vi "ControlClass.vi"(7 "PythonConverter_GUI in":refnum<class "PythonConverter_GUI.lvclass">, 8 "error in":errorcluster, 11 "Control in":refnum<class "Control.lvclass">) -> (0 "error out":errorcluster, 3 "Control out":refnum<class "Control.lvclass">, 4 "control name":string, 5 "PythonConverter_GUI out":refnum<class "PythonConverter_GUI.lvclass">)   [LabVIEW 2014, in "Raspberry Pi Compatible Compiler for LabVIEW.lvlib" / "PythonConverter_GUI.lvclass"]
uses:
  PythonConverter_GUI.lvclass
  VI Interpreter/Classes/Control/Control.lvclass
  VI Interpreter/Classes/NumericWithScale/NumericWithScale.lvclass/NumericWithScale.ctl
  Parsing/ClassTypeTD.ctl
  VI Interpreter/Classes/Control/Control.lvclass/Control.ctl
  VI Interpreter/Classes/Digital/Digital.lvclass
  VI Interpreter/Classes/Tab/Tab.lvclass
  VI Interpreter/Classes/Cluster/Cluster.lvclass
  VI Interpreter/Classes/Knob/Knob.lvclass
  VI Interpreter/Classes/Slide/Slide.lvclass
  VI Interpreter/Classes/Ring/Ring.lvclass
  VI Interpreter/Classes/Enum/Enum.lvclass
  VI Interpreter/Classes/NumericWithScale/NumericWithScale.lvclass
  Parsing/Python Functions.lvlib
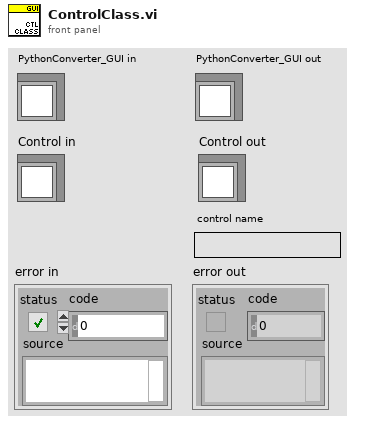
[diagram p1: front panel]
types:
  T1 = typedef "Raspberry Pi Compatible Compiler for LabVIEW.lvlib/Python Functions.lvlib/ClassTypeTD.ctl" = enum16{"class", "function"}
  T2 = typedef "Raspberry Pi Compatible Compiler for LabVIEW.lvlib/PythonConverter_GUI.lvclass/FPOwnerClassTD.ctl" = enum16{"Panel", "Array", "Cluster", "Tab control"}
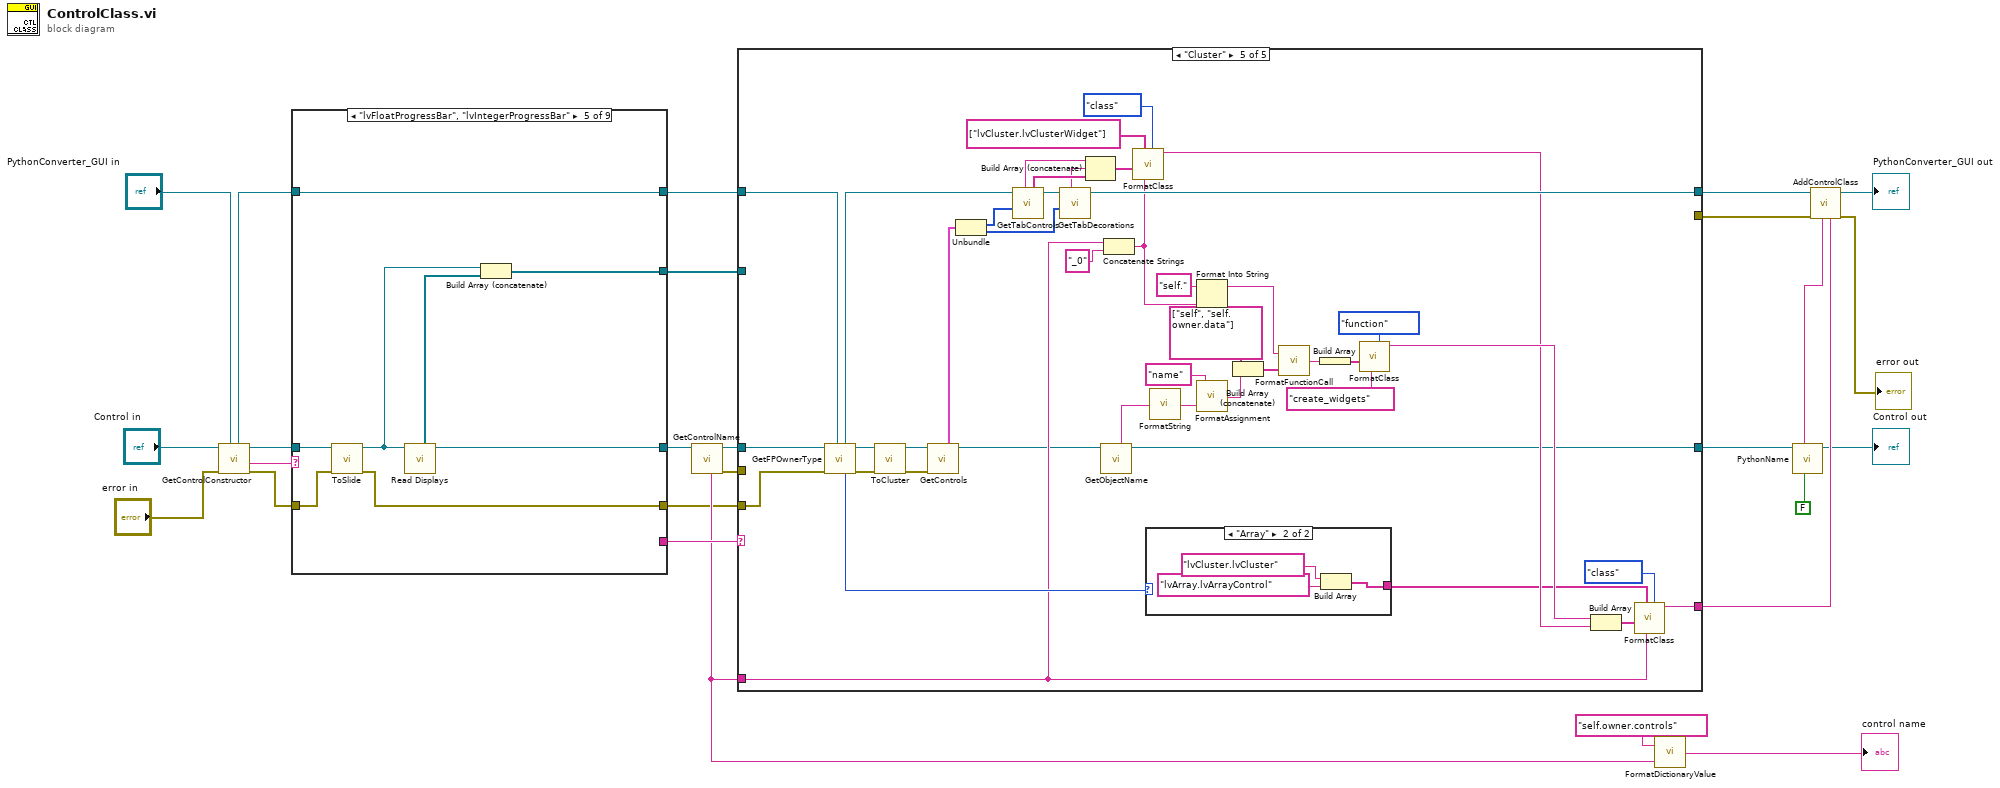
[diagram p0: block diagram]
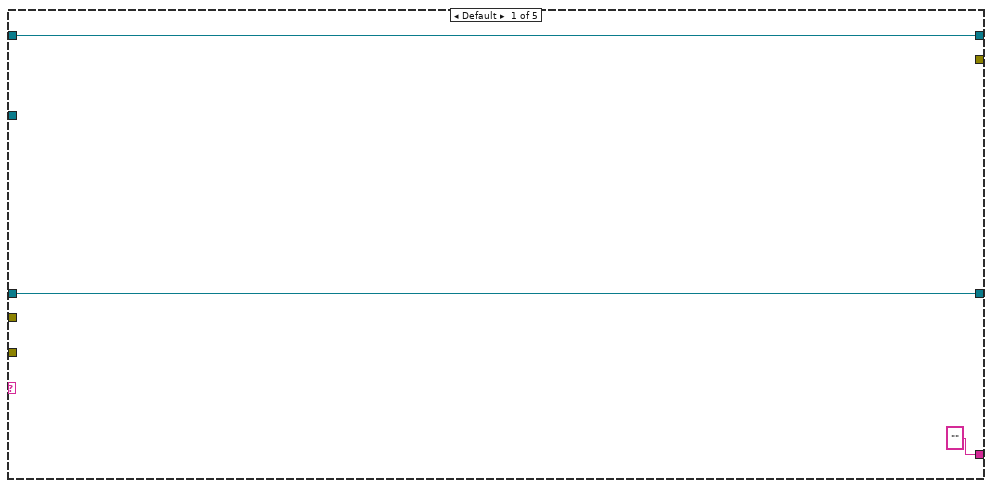
[diagram p2: hidden frame]
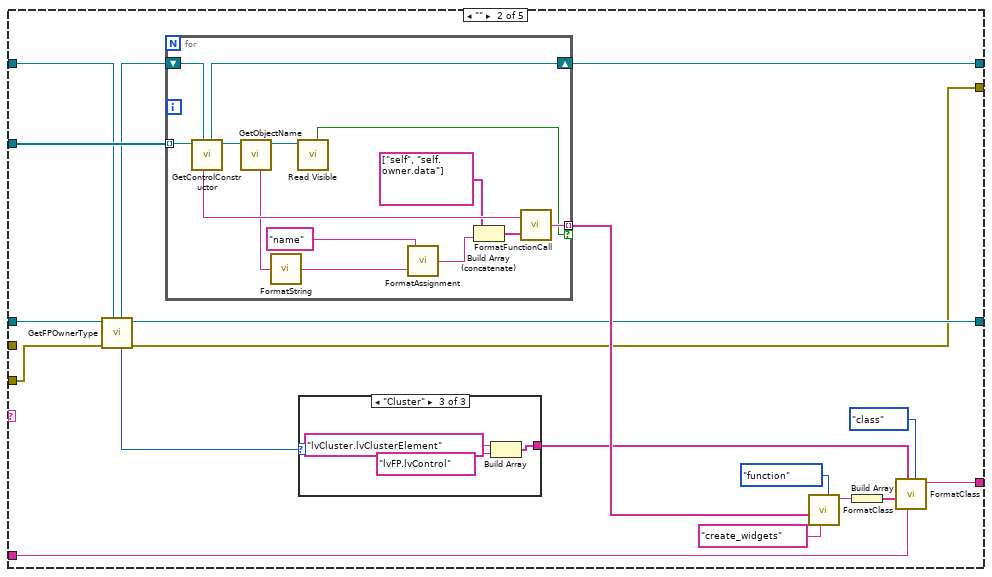
[diagram p3: hidden frame]
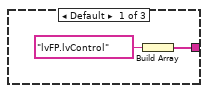
[diagram p4: hidden frame]
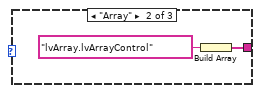
[diagram p5: hidden frame]
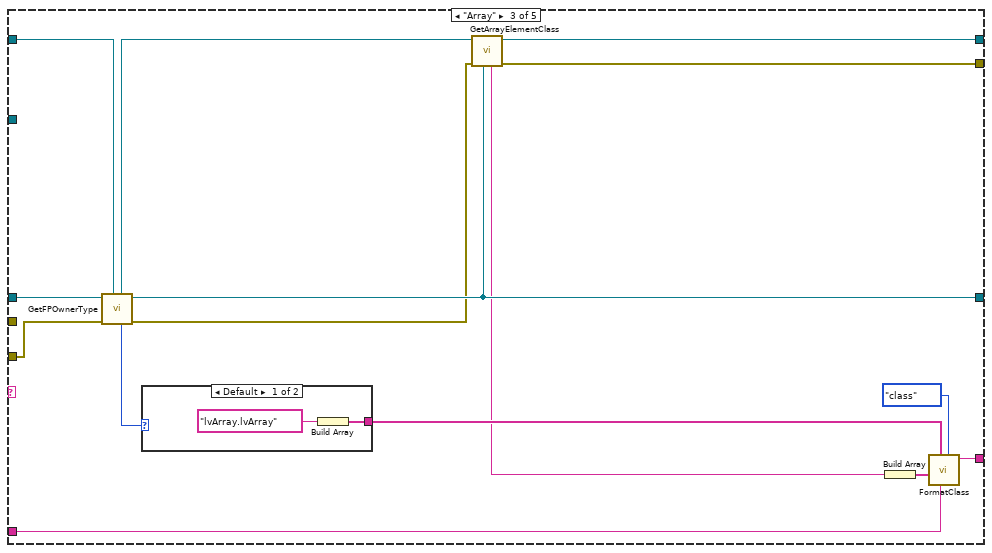
[diagram p6: hidden frame]
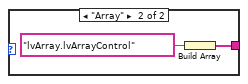
[diagram p7: hidden frame]
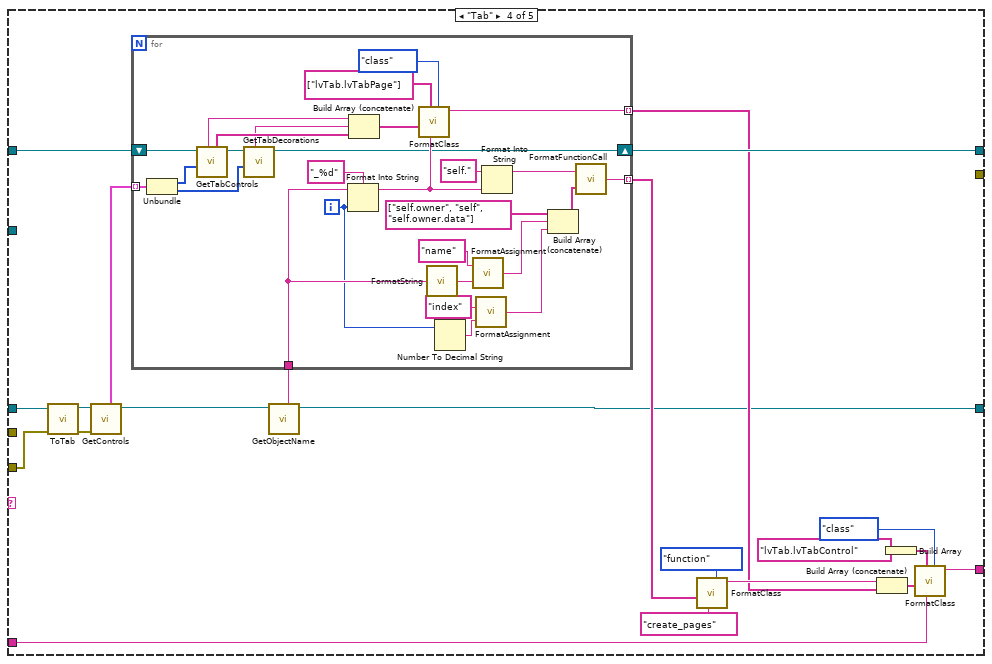
[diagram p8: hidden frame]
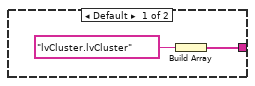
[diagram p9: hidden frame]
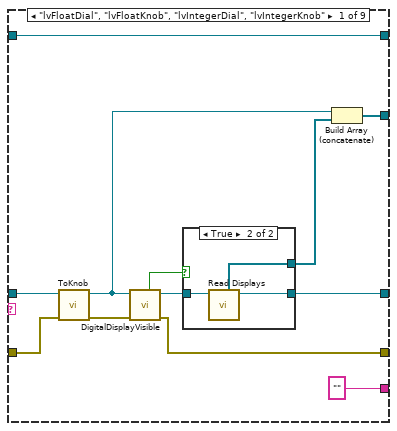
[diagram p10: hidden frame]
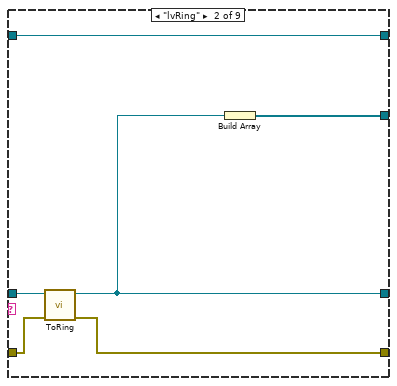
[diagram p12: hidden frame]
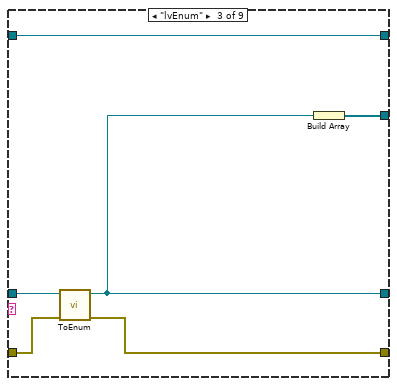
[diagram p13: hidden frame]
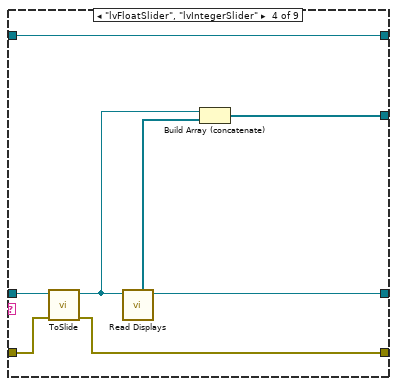
[diagram p14: hidden frame]
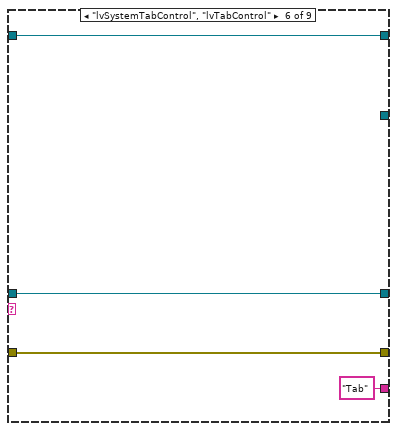
[diagram p15: hidden frame]
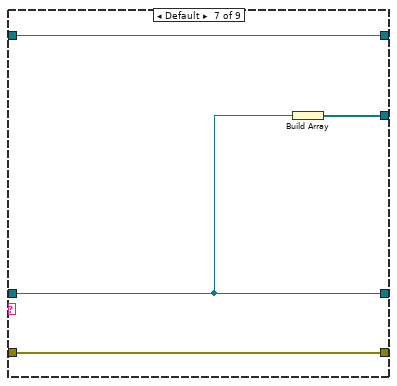
[diagram p16: hidden frame]
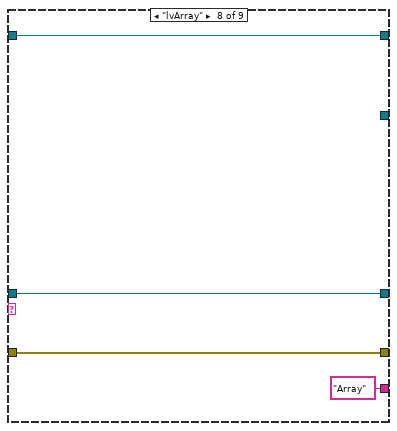
[diagram p17: hidden frame]
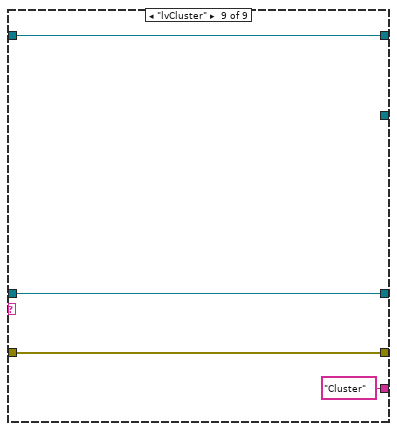
[diagram p18: hidden frame]
diagram:
  n1 = call "GetControlConstructor.vi"("PythonConverter_GUI in"="PythonConverter_GUI in", "error in"="error in", "Control in"="Control in") -> ("error out"=w21:errorcluster, "class"=w15:string, "Control out"=w25:refnum<class "Control.lvclass">, "PythonConverter_GUI out"=w2:refnum<class "PythonConverter_GUI.lvclass">)  [unwired: 2 in, 3 out]
  n2 = case shown="\"lvFloatProgressBar\", \"lvIntegerProgressBar\"" w15 {
    tunnel: w25 -> [w38 w48 w54 w62 w70 w71 w76 w79 w83]
    tunnel: [w37 w45 w51 w59 w67 w71 w76 w79 w83] -> w8
    tunnel: [w33 w44 w50 w57 w65 _ w75 _ _] -> w23
    tunnel: w21 -> [w35 w47 w53 w61 w69 w72 w78 w80 w84]
    tunnel: [w30 w46 w52 w58 w66 w72 w78 w80 w84] -> w5
    tunnel: ["" ("format string") _ _ _ _ "Tab" ("format string") _ "Array" ("format string") "Cluster" ("format string")] -> w18
    tunnel: w2 -> [w27 w43 w49 w55 w63 w74 w77 w81 w85]
    tunnel: [w27 w43 w49 w55 w63 w74 w77 w81 w85] -> w1
    frame "lvFloatDial", "lvFloatKnob", "lvIntegerDial", "lvIntegerKnob" {
      n3 = call "ToKnob.vi"("error in"=w35, "Generic"=w38) -> ("error out"=w31:errorcluster, "Knob out"=w32:refnum<class "Knob.lvclass">)  [unwired: 8 in]
      n4 = call "DigitalDisplayVisible.vi"("error in"=w31, "Knob in"=w32) -> ("error out"=w30:errorcluster, "Knob out"=w29:refnum<class "Knob.lvclass">, "digital display"=w28:bool)  [unwired: 5 in]
      n5 = case shown="True" w28 {
        tunnel: [w39 w42] -> w37
        tunnel: [_ w41] -> w36
        tunnel: w29 -> [w39 w40]
        frame False {
        }
        frame True {
          n6 = call "Read Displays.vi"("NumericWithScale in"=w40) -> ("NumericWithScale out"=w42:refnum<class "Knob.lvclass">, "Displays"=w41:refnum<class "Digital.lvclass">[])  [unwired: 7 in]
        }
      }
      n7 = Build Array (concatenate)(w32, w36) -> (w33:refnum<class "Numeric.lvclass">[])
    }
    frame "lvRing" {
      n8 = call "ToRing.vi"("error in"=w47, "Ring in"=w48) -> ("error out"=w46:errorcluster, "Ring out"=w45:refnum<class "Ring.lvclass">)  [unwired: 8 in]
      n9 = Build Array(w45) -> (w44:refnum<class "Ring.lvclass">[])
    }
    frame "lvEnum" {
      n10 = call "ToEnum.vi"("error in"=w53, "Ring in"=w54) -> ("error out"=w52:errorcluster, "Enum out"=w51:refnum<class "Enum.lvclass">)  [unwired: 8 in]
      n11 = Build Array(w51) -> (w50:refnum<class "Enum.lvclass">[])
    }
    frame "lvFloatSlider", "lvIntegerSlider" {
      n12 = call "ToSlide.vi"("error in"=w61, "Generic"=w62) -> ("error out"=w58:errorcluster, "Slide out"=w56:refnum<class "Slide.lvclass">)  [unwired: 8 in]
      n13 = call "Read Displays.vi"("NumericWithScale in"=w56) -> ("NumericWithScale out"=w59:refnum<class "Slide.lvclass">, "Displays"=w60:refnum<class "Digital.lvclass">[])  [unwired: 7 in]
      n14 = Build Array (concatenate)(w56, w60) -> (w57:refnum<class "Numeric.lvclass">[])
    }
    frame "lvFloatProgressBar", "lvIntegerProgressBar" {
      n15 = call "ToSlide.vi"("error in"=w69, "Generic"=w70) -> ("error out"=w66:errorcluster, "Slide out"=w64:refnum<class "Slide.lvclass">)  [unwired: 8 in]
      n16 = call "Read Displays.vi"("NumericWithScale in"=w64) -> ("NumericWithScale out"=w67:refnum<class "Slide.lvclass">, "Displays"=w68:refnum<class "Digital.lvclass">[])  [unwired: 7 in]
      n17 = Build Array (concatenate)(w64, w68) -> (w65:refnum<class "Numeric.lvclass">[])
    }
    frame "lvSystemTabControl", "lvTabControl" {
    }
    frame Default {
      n18 = Build Array(w76) -> (w75:refnum<class "Control.lvclass">[])
    }
    frame "lvArray" {
    }
    frame "lvCluster" {
    }
  }
  n19 = call "GetControlName.vi"("Control in"=w8) -> ("error out"=w3:errorcluster, "Control out"=w7:refnum<class "Control.lvclass">, "name"=w6:string)  [unwired: 6 in]
  n20 = case shown="\"Cluster\"" w18 {
    tunnel: w1 -> [w89 w94 w138 w153 w225]
    tunnel: w23 -> [_ w107 _ _ _]
    tunnel: [w89 w106 w134 w152 w239] -> w22
    tunnel: ["" ("python") w105 w143 w168 w219] -> w20
    tunnel: w7 -> [w87 w97 w135 w165 w226]
    tunnel: [w87 w96 w133 w149 w198] -> w12
    tunnel: w6 -> [_ w98 w140 w159 w204]
    tunnel: w5 -> [_ w92 w137 w164 w223]
    tunnel: [_ w91 w132 _ _] -> w4
    tunnel: w3 -> [_ _ _ _ _]
    frame Default {
    }
    frame "" {
      n21 = call "GetFPOwnerType.vi"("PythonConverter_GUI in"=w94, "error in"=w92, "Object in"=w97) -> ("error out"=w91:errorcluster, "Object out"=w96:refnum<class "Control.lvclass">, "owner"=w95:T2, "PythonConverter_GUI out"=w93:refnum<class "PythonConverter_GUI.lvclass">)  [unwired: 5 in]
      n22 = for {
        shift-right: [w117] -> w106
        shift-left: w93 -> [w128]
        tunnel: w107 -> [w127] mode=indexing
        tunnel: [w125] -> w99 mode=indexing if=w115
        n23 = call "GetControlConstructor.vi"("PythonConverter_GUI in"=w128, "Control in"=w127) -> ("Control out"=w119:refnum<class "Control.lvclass">, "PythonConverter_GUI out"=w117:refnum<class "PythonConverter_GUI.lvclass">, "constructor"=w126:string)  [unwired: 3 in, 4 out]
        n24 = call-dynamic "GetObjectName.vi"("GObject in"=w119) -> ("GObject out"=w116:refnum<class "Control.lvclass">, "Name"=w118:string)  [unwired: 6 in, 1 out]
        n25 = call "FormatString.vi"("value"=w118) -> ("python object"=w124:string)
        n26 = call "Read Visible.vi"("Control in"=w116) -> ("Visible"=w115:bool)  [unwired: 7 in, 1 out]
        n27 = call "FormatAssignment.vi"("value"=w124, "name"="name") -> ("python assignment"=w122:string)
        n28 = Build Array (concatenate)(string[] ["self", "self.owner.data"] ("appended array"), w122) -> (w121:string[])
        n29 = call "FormatFunctionCall.vi"("parameters"=w121, "function"=w126) -> ("python object"=w125:string)
      }
      n30 = case shown="\"Cluster\"" w95 {
        tunnel: [w108 w110 w113] -> w90
        frame Default {
          n31 = Build Array("lvFP.lvControl" ("format string")) -> (w108:string[])
        }
        frame "Array" {
          n32 = Build Array("lvArray.lvArrayControl" ("format string")) -> (w110:string[])
        }
        frame "Cluster" {
          n33 = Build Array("lvCluster.lvClusterElement" ("format string"), "lvFP.lvControl" ("format string")) -> (w113:string[])
        }
      }
      n34 = call "FormatClass.vi"("type"=ClassTypeTD."function", "name"="create_widgets", "body"=w99) -> ("python"=w102:string)  [unwired: 8 in]
      n35 = Build Array(w102) -> (w101:string[])
      n36 = call "FormatClass.vi"("type"=ClassTypeTD."class", "name"=w98, "parameters/ancestors"=w90, "body"=w101) -> ("python"=w105:string)  [unwired: 7 in]
    }
    frame "Array" {
      n37 = call "GetFPOwnerType.vi"("PythonConverter_GUI in"=w138, "error in"=w137, "Object in"=w135) -> ("error out"=w131:errorcluster, "Object out"=w133:refnum<class "Control.lvclass">, "owner"=w139:T2, "PythonConverter_GUI out"=w129:refnum<class "PythonConverter_GUI.lvclass">)  [unwired: 5 in]
      n38 = case shown="Default" w139 {
        tunnel: [w144 w146] -> w136
        frame Default {
          n39 = Build Array("lvArray.lvArray" ("format string")) -> (w144:string[])
        }
        frame "Array" {
          n40 = Build Array("lvArray.lvArrayControl" ("format string")) -> (w146:string[])
        }
      }
      n41 = call "GetArrayElementClass.vi"("Control in"=w133, "error in"=w131, "PythonConverter_GUI in"=w129) -> ("error out"=w132:errorcluster, "PythonConverter_GUI out"=w134:refnum<class "PythonConverter_GUI.lvclass">, "class"=w130:string)  [unwired: 4 in]
      n42 = Build Array(w130) -> (w141:string[])
      n43 = call "FormatClass.vi"("type"=ClassTypeTD."class", "name"=w140, "parameters/ancestors"=w136, "body"=w141) -> ("python"=w143:string)  [unwired: 7 in]
    }
    frame "Tab" {
      n44 = call "ToTab.vi"("error in"=w164, "Generic in"=w165) -> ("error out"=w161:errorcluster, "Tab out"=w162:refnum<class "Tab.lvclass">)  [unwired: 8 in]
      n45 = call "GetControls.vi"("error in"=w161, "Tab in"=w162) -> ("Tab out"=w150:refnum<class "Tab.lvclass">, "Controls"=w160:cluster{"controls":i32[], "decorations":i32[]}[])  [unwired: 5 in, 1 out]
      n46 = call-dynamic "GetObjectName.vi"("GObject in"=w150) -> ("GObject out"=w149:refnum<class "Tab.lvclass">, "Name"=w148:string)  [unwired: 6 in, 1 out]
      n47 = for {
        tunnel: w160 -> [w196] mode=indexing
        shift-right: [w171] -> w152
        shift-left: w153 -> [w194]
        tunnel: w148 -> [w181]
        tunnel: [w189] -> w151 mode=indexing
        tunnel: [w175] -> w156 mode=indexing
        i -> [w176]
        n48 = Unbundle(w196) -> ("controls"=w195:i32[], "decorations"=w172:i32[])
        n49 = call "GetTabControls.vi"("controls"=w195, "PythonConverter_GUI in"=w194) -> ("PythonConverter_GUI out"=w173:refnum<class "PythonConverter_GUI.lvclass">, "classes"=w174:string[], "create_controls"=w170:string)  [unwired: 5 in]
        n50 = call "GetTabDecorations.vi"("decorations"=w172, "PythonConverter_GUI in"=w173) -> ("PythonConverter_GUI out"=w171:refnum<class "PythonConverter_GUI.lvclass">, "create_decorations"=w169:string)  [unwired: 6 in]
        n51 = Format Into String(format string="_%d", initial string=w181, w176) -> (resulting string=w187:string)  [unwired: 1 in, 1 out]
        n52 = Build Array (concatenate)(w170, w169, w174) -> (w190:string[])
        n53 = call "FormatClass.vi"("type"=ClassTypeTD."class", "name"=w187, "parameters/ancestors"=string[] ["lvTab.lvTabPage"], "body"=w190) -> ("python"=w189:string)  [unwired: 7 in]
        n54 = call "FormatString.vi"("value"=w181) -> ("python object"=w182:string)
        n55 = Number To Decimal String(number=w176) -> (decimal integer string=w177:string)  [unwired: 1 in]
        n56 = call "FormatAssignment.vi"("value"=w182, "name"="name") -> ("python assignment"=w180:string)
        n57 = call "FormatAssignment.vi"("value"=w177, "name"="index") -> ("python assignment"=w178:string)
        n58 = Format Into String(initial string="self.", w187) -> (resulting string=w186:string)  [unwired: 2 in, 1 out]
        n59 = Build Array (concatenate)(string[] ["self.owner", "self", "self.owner.data"] ("appended array"), w180, w178) -> (w185:string[])
        n60 = call "FormatFunctionCall.vi"("parameters"=w185, "function"=w186) -> ("python object"=w175:string)
      }
      n61 = call "FormatClass.vi"("type"=ClassTypeTD."function", "name"="create_pages", "body"=w156) -> ("python"=w157:string)  [unwired: 8 in]
      n62 = Build Array (concatenate)(w157, w151) -> (w158:string[])
      n63 = Build Array("lvTab.lvTabControl" ("format string")) -> (w166:string[])
      n64 = call "FormatClass.vi"("type"=ClassTypeTD."class", "name"=w159, "parameters/ancestors"=w166, "body"=w158) -> ("python"=w168:string)  [unwired: 7 in]
    }
    frame "Cluster" {
      n65 = call "GetFPOwnerType.vi"("PythonConverter_GUI in"=w225, "error in"=w223, "Object in"=w226) -> ("error out"=w227:errorcluster, "Object out"=w228:refnum<class "Control.lvclass">, "owner"=w222:T2, "PythonConverter_GUI out"=w224:refnum<class "PythonConverter_GUI.lvclass">)  [unwired: 5 in]
      n66 = call "ToCluster.vi"("error in"=w227, "Generic"=w228) -> ("error out"=w221:errorcluster, "Cluster out"=w238:refnum<class "Cluster.lvclass">)  [unwired: 8 in]
      n67 = call "GetControls.vi"("error in"=w221, "Cluster in"=w238) -> ("Cluster in"=w200:refnum<class "Cluster.lvclass">, "controls"=w229:cluster{"controls":i32[], "decorations":i32[]})  [unwired: 5 in, 1 out]
      n68 = Unbundle(w229) -> ("controls"=w237:i32[], "decorations"=w232:i32[])
      n69 = call "GetTabControls.vi"("controls"=w237, "PythonConverter_GUI in"=w224) -> ("PythonConverter_GUI out"=w233:refnum<class "PythonConverter_GUI.lvclass">, "classes"=w234:string[], "create_controls"=w231:string)  [unwired: 5 in]
      n70 = call "GetTabDecorations.vi"("decorations"=w232, "PythonConverter_GUI in"=w233) -> ("PythonConverter_GUI out"=w239:refnum<class "PythonConverter_GUI.lvclass">, "create_decorations"=w230:string)  [unwired: 6 in]
      n71 = Build Array (concatenate)(w231, w230, w234) -> (w235:string[])
      n72 = call-dynamic "GetObjectName.vi"("GObject in"=w200) -> ("GObject out"=w198:refnum<class "Cluster.lvclass">, "Name"=w199:string)  [unwired: 6 in, 1 out]
      n73 = Concatenate Strings(w204, "_0" ("string")) -> (w201:string)
      n74 = call "FormatClass.vi"("type"=ClassTypeTD."class", "name"=w201, "parameters/ancestors"=string[] ["lvCluster.lvClusterWidget"], "body"=w235) -> ("python"=w205:string)  [unwired: 7 in]
      n75 = case shown="\"Array\"" w222 {
        tunnel: [w240 w243] -> w197
        frame Default {
          n76 = Build Array("lvCluster.lvCluster" ("format string")) -> (w240:string[])
        }
        frame "Array" {
          n77 = Build Array("lvCluster.lvCluster" ("format string"), "lvArray.lvArrayControl" ("format string")) -> (w243:string[])
        }
      }
      n78 = call "FormatString.vi"("value"=w199) -> ("python object"=w212:string)
      n79 = Format Into String(initial string="self.", w201) -> (resulting string=w203:string)  [unwired: 2 in, 1 out]
      n80 = call "FormatAssignment.vi"("value"=w212, "name"="name") -> ("python assignment"=w210:string)
      n81 = Build Array (concatenate)(string[] ["self", "self.owner.data"] ("appended array"), w210) -> (w209:string[])
      n82 = call "FormatFunctionCall.vi"("parameters"=w209, "function"=w203) -> ("python object"=w207:string)
      n83 = Build Array(w207) -> (w206:string[])
      n84 = call "FormatClass.vi"("type"=ClassTypeTD."function", "name"="create_widgets", "body"=w206) -> ("python"=w215:string)  [unwired: 8 in]
      n85 = Build Array(w215, w205) -> (w214:string[])
      n86 = call "FormatClass.vi"("type"=ClassTypeTD."class", "name"=w204, "parameters/ancestors"=w197, "body"=w214) -> ("python"=w219:string)  [unwired: 7 in]
    }
  }
  n87 = call "FormatDictionaryValue.vi"("key"=w6, "dictionary"="self.owner.controls") -> ("python object"=→"control name":string)
  n88 = call-dynamic "PythonName.vi"("add self"=FALSE, "GObject in"=w12) -> ("GObject out"=→"Control out":refnum<class "Control.lvclass">, "UID"=w16:string)  [unwired: 6 in, 2 out]
  n89 = call "AddControlClass.vi"("class"=w20, "name"=w16, "error in"=w4, "PythonConverter_GUI in"=w22) -> ("error out"=→"error out":errorcluster, "PythonConverter_GUI out"=→"PythonConverter_GUI out":refnum<class "PythonConverter_GUI.lvclass">)  [unwired: 4 in]
